vi "Transient Capture - Configure Settings.vi"(7 "Soft Trigger":bool=TRUE, 8 "error in":errorcluster, 9 "Samples to Read (Post Trigger)":i32=100000, 10 "Samples to Read (Pre Trigger)":i32=100000, 11 "Address":string) -> (0 "error out":errorcluster, 1 "AI Connection Out":T1={"Description"="", "Address"="", "Port"=0, "timeout (ms)"=5000, "Termination Character"="\n", "TCP Connection Reference"=refnum, "Open Connection"=FALSE}, 2 "Carrier Connection Out":T1={"Description"="", "Address"="", "Port"=0, "timeout (ms)"=5000, "Termination Character"="\n", "TCP Connection Reference"=refnum, "Open Connection"=FALSE})   [LabVIEW 2017, in "Communications Library.lvlib"]
doc: "Configures the DTACQ device for transient capture mode.\n\nSets the transient capture mode, trigger mode and event settings."
uses:
  Communications Library.lvlib
  Typedefs/DTACQ Connection Data--Cluster.ctl
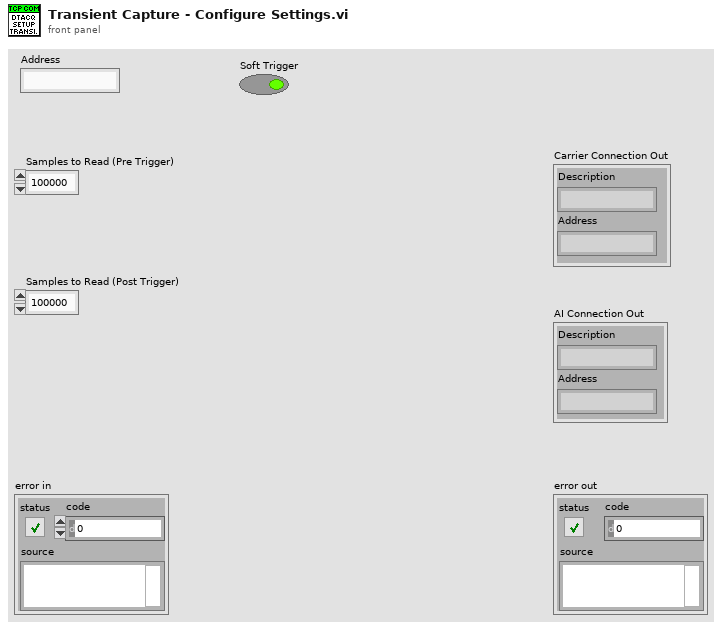
[diagram p1: front panel]
types:
  T1 = typedef "Communications Library.lvlib/DTACQ Connection Data--Cluster.ctl" = cluster{"Description":string, "Address":string, "Port":u16, "timeout (ms)":i32, "Termination Character":string, "TCP Connection Reference":refnum<k5>, "Open Connection":bool}
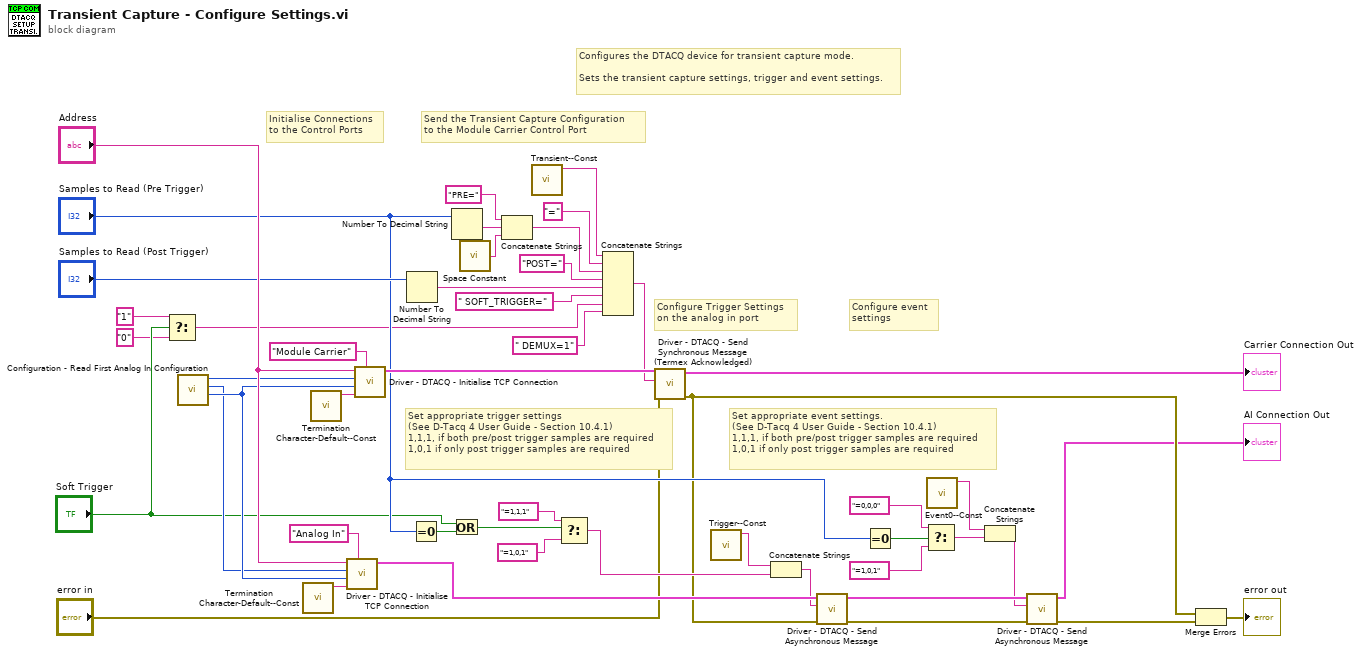
[diagram p0: block diagram]
diagram:
  # "Configure event\nsettings"
  # "Set appropriate event settings.\n(See D-Tacq 4 User Guide - Section 10.4.1)\n1,1,1, if both pre/post trigger samples are required\n1,0,1 if only post trigger samples are required"
  # "Set appropriate trigger settings\n(See D-Tacq 4 User Guide - Section 10.4.1)\n1,1,1, if both pre/post trigger samples are required\n1,0,1 if only post trigger samples are required"
  # "Configures the DTACQ device for transient capture mode.\n\nSets the transient capture settings, trigger and event settings."
  # "Configure Trigger Settings\non the analog in port"
  # "Send the Transient Capture Configuration\nto the Module Carrier Control Port"
  # "Initialise Connections\nto the Control Ports"
  n1 = Select(t="1", s="Soft Trigger", f="0") -> (s? t:f=w2:string)
  n2 = call "Configuration - Read First Analog In Configuration.vi"() -> ("Timeout (ms)"=w16:i32, "Analog In Control Port"=w15:i32, "Carrier Control Port"=w34:i32)  [unwired: 7 in, 2 out]
  n3 = call "Termination Character-Default--Const.vi"() -> ("Termination Character"=w42:string)  [unwired: 11 in]
  n4 = call "Termination Character-Default--Const.vi"() -> ("Termination Character"=w44:string)  [unwired: 11 in]
  n5 = call "Driver - DTACQ - Initialise TCP Connection.vi"("Description"="Analog In", "Termination Character"=w42, "timeout (ms)"=w16, "Port"=w15, "Address"="Address") -> ("DTACQ Connection Data Out"=w47:T1)  [unwired: 6 in]
  n6 = call "Driver - DTACQ - Initialise TCP Connection.vi"("Description"="Module Carrier", "Termination Character"=w44, "timeout (ms)"=w16, "Port"=w34, "Address"="Address") -> ("DTACQ Connection Data Out"=w36:T1)  [unwired: 6 in]
  n7 = Number To Decimal String(number="Samples to Read (Post Trigger)") -> (decimal integer string=w41:string)  [unwired: 1 in]
  n8 = Equal To 0?(x="Samples to Read (Pre Trigger)") -> (x = 0?=w13:bool)
  n9 = Number To Decimal String(number="Samples to Read (Pre Trigger)") -> (decimal integer string=w29:string)  [unwired: 1 in]
  n10 = Or(x="Soft Trigger", y=w13) -> (x .or. y?=w12:bool)
  n11 = call <vilib>:"Space Constant.vi"() -> ("String"=w28:string)
  n12 = Concatenate Strings("PRE=" ("string"), w29, w28) -> (w31:string)
  n13 = call "Transient--Const.vi"() -> ("Transient Command"=w33:string)  [unwired: 11 in]
  n14 = Select(t="=1,1,1" ("string"), s=w12, f="=1,0,1" ("string")) -> (s? t:f=w27:string)
  n15 = Concatenate Strings(w33, "=" ("string"), w31, "POST=" ("string"), w41, " SOFT_TRIGGER=" ("string"), w2, " DEMUX=1") -> (w35:string)
  n16 = call "Driver - DTACQ - Send Synchronous Message (Termex Acknowledged).vi"("error in"="error in", "Message to Send"=w35, "DTACQ Connection Data In"=w36) -> ("error out"=w9:errorcluster, "DTACQ Connection Data Out"=→"Carrier Connection Out":T1)  [unwired: 5 in, 2 out]
  n17 = call "Trigger--Const.vi"() -> ("Trigger Command"=w38:string)  [unwired: 11 in]
  n18 = Concatenate Strings(w38, w27) -> (w37:string)
  n19 = call "Driver - DTACQ - Send Asynchronous Message.vi"("error in"=w9, "Message to Send"=w37, "DTACQ Connection Data In"=w47) -> ("error out"=w21:errorcluster, "DTACQ Connection Data Out"=w22:T1)  [unwired: 7 in]
  n20 = Equal To 0?(x="Samples to Read (Pre Trigger)") -> (x = 0?=w19:bool)
  n21 = Select(t="=0,0,0" ("string"), s=w19, f="=1,0,1" ("string")) -> (s? t:f=w23:string)
  n22 = call "Event0--Const.vi"() -> ("Event Command"=w26:string)  [unwired: 11 in]
  n23 = Concatenate Strings(w26, w23) -> (w18:string)
  n24 = call "Driver - DTACQ - Send Asynchronous Message.vi"("error in"=w21, "Message to Send"=w18, "DTACQ Connection Data In"=w22) -> ("error out"=w7:errorcluster, "DTACQ Connection Data Out"=→"AI Connection Out":T1)  [unwired: 7 in]
  n25 = Merge Errors(w9, w7) -> (→"error out":errorcluster)
